vi "test Endpoint Configurations.vi"(8 "error in (no error)":errorcluster, 11 "TestCase in":refnum<class "SLSC Switch Scripting Unit Tests.lvclass">) -> (0 "error out":errorcluster, 3 "TestCase out":refnum<class "SLSC Switch Scripting Unit Tests.lvclass">)   [LabVIEW 2017, in "SLSC Switch Scripting Unit Tests.lvclass"]
uses:
  SLSC Switch Scripting Unit Tests.lvclass
  Endpoint Configuration/Endpoint Configuration Enum.ctl
  SLSC Switch Scripting Unit Tests.lvclass/SLSC Switch Scripting Unit Tests.ctl
  <vilib>/addons/_JKI Toolkits/VI Tester/TestCase.llb/TestCase.lvclass
  SLSC Switch Scripting.lvlib
  C:/Program Files (x86)/National Instruments/LabVIEW 2017/vi.lib/addons/_JKI Toolkits/VI Tester/TestCase.llb/TestCase.lvclass
panel:
  in  "Save?":bool
  out "Output Filename":string
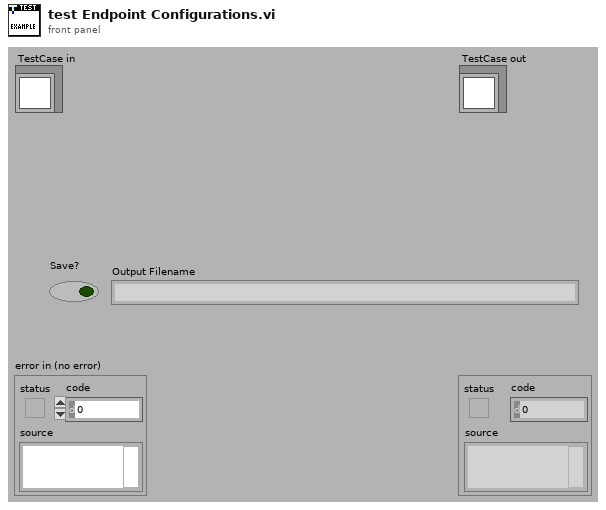
[diagram p1: front panel]
types:
  T1 = typedef "SLSC Switch Scripting.lvlib/Endpoint Configuration Enum.ctl" = enum16{"Load", "Source", "Configuration"}
  T2 = typedef "Custom Device API.lvlib/Custom Device Item Ref.ctl" = u64
  T3 = typedef "SLSC Switch Scripting.lvlib/Endpoint Configuration Cluster.ctl" = cluster{"endpoint":string, "configuration":T1}
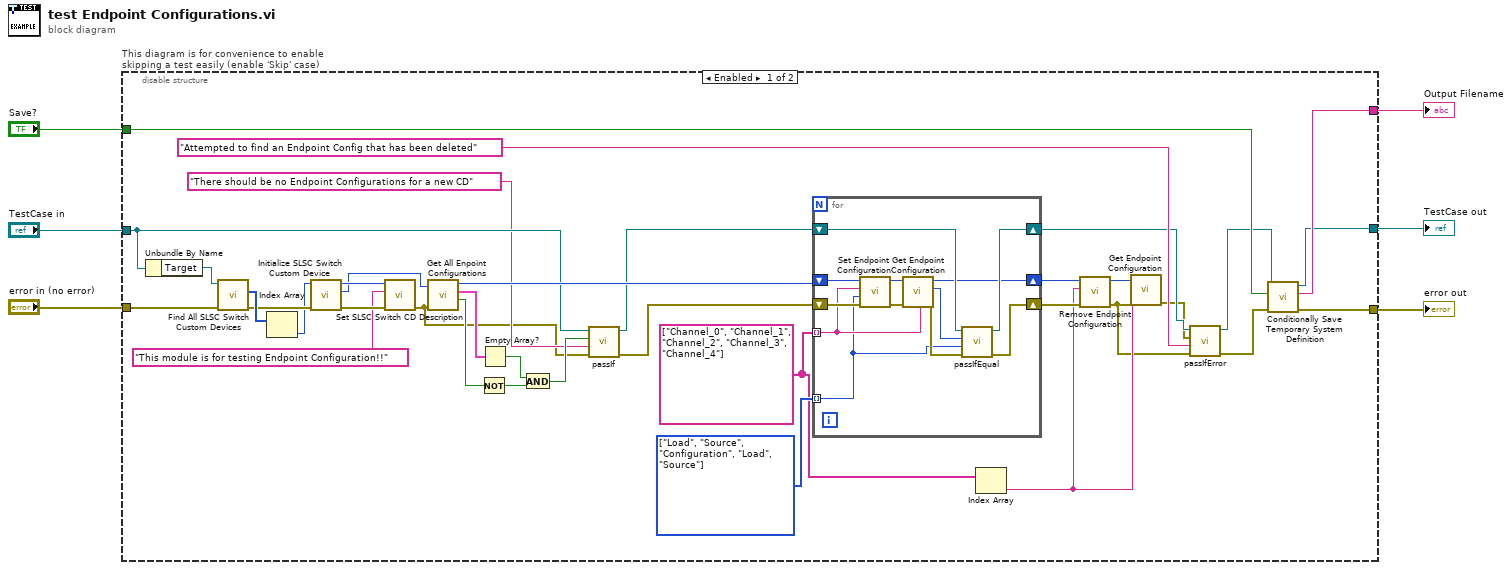
[diagram p0: block diagram]
diagram:
  n1 = disable-structure "This diagram is for convenience to enable skipping a test easily (enable 'Skip' case)" shown="Enabled" {
    disable-tunnel: "TestCase in" -> [w22 w58]
    disable-tunnel: [w40 w56] -> w3
    disable-tunnel: [w41 w57] -> w5
    disable-tunnel: "error in (no error)" -> [w34 w55]
    disable-tunnel: [w42 _] -> w2
    disable-tunnel: "Save?" -> [w39 _]
    frame Enabled {
      w16 = string[] ["Channel_0", "Channel_1", "Channel_2", "Channel_3", "Channel_4"]
      w30 = T1[] [enum."Load", enum."Source", enum."Configuration", enum."Load", enum."Source"] items=["Load", "Source", "Configuration"]
      n2 = Unbundle By Name(w22) -> ("Target"=w35:refnum<k24>)
      n3 = call "Find All SLSC Switch Custom Devices.vi"("error in (no error)"=w34, "Target in"=w35) -> ("error out"=w37:errorcluster, "SLSC Switch Custom Device Ref IDs"=w38:T2[])  [unwired: 7 in, 1 out]
      n4 = Index Array(array=w38) -> (element=w36:T2)  [unwired: 1 in]
      n5 = call "Initialize SLSC Switch Custom Device.vi"("error in (no error)"=w37, "SLSC Sw Custom Device Ref in"=w36) -> ("error out"=w32:errorcluster, "Endpoint Configuration Section Ref"=w29:T2, "SLSC Sw Custom Device Ref out"=w33:T2)  [unwired: 7 in]
      n6 = call "Set SLSC Switch CD Description.vi"("error in (no error)"=w32, "Description"="This module is for testing Endpoint Configuration!!", "SLSC Sw Custom Device Ref in"=w33) -> ("error out"=w18:errorcluster)  [unwired: 7 in, 1 out]
      n7 = call "Get All Enpoint Configurations.vi"("error in (no error)"=w18, "Endpoint Config Section Ref in"=w29) -> ("Endpoints found"=w24:bool, "All Endpoint Configurations"=w27:T3[], "Endpoint Config Section Ref out"=w28:T2)  [unwired: 6 in, 1 out]
      n8 = Not(x=w24) -> (.not. x?=w25:bool)
      n9 = Empty Array?(array=w27) -> (empty?=w26:bool)
      n10 = And(x=w26, y=w25) -> (x .and. y?=w23:bool)
      n11 = call-dynamic "passIf.vi"("error in (no error)"=w18, "message (\"\")"="There should be no Endpoint Configurations for a new CD" ("message (\"\")"), "pass"=w23, "TestCase in"=w22) -> ("error out"=w19:errorcluster, "TestCase out"=w21:refnum<class "SLSC Switch Scripting Unit Tests.lvclass">)  [unwired: 6 in]
      n12 = for {
        shift-right: [w47] -> w15
        shift-left: w19 -> [w53]
        shift-right: [w49] -> w11
        shift-left: w21 -> [w50]
        tunnel: w16 -> [w46] mode=indexing
        tunnel: w30 -> [w43] mode=indexing
        shift-right: [w45] -> w17
        shift-left: w28 -> [w54]
        n13 = call "Set Endpoint Configuration.vi"("error in (no error)"=w53, "Configuration Type"=w43, "Endpoint"=w46, "Endpoint Config Section Ref in"=w54) -> ("error out"=w51:errorcluster, "Endpoint Config Section Ref in"=w52:T2)  [unwired: 6 in]
        n14 = call "Get Endpoint Configuration.vi"("error in (no error)"=w51, "Endpoint"=w46, "Endpoint Config Section Ref in"=w52) -> ("error out"=w48:errorcluster, "Configuration Type"=w44:T1, "Endpoint Config Section Ref out"=w45:T2)  [unwired: 5 in, 1 out]
        n15 = call-dynamic "passIfEqual.vi"("error in (no error)"=w48, "y"=w43, "x"=w44, "TestCase in"=w50) -> ("error out"=w47:errorcluster, "TestCase out"=w49:refnum<class "SLSC Switch Scripting Unit Tests.lvclass">)  [unwired: 6 in]
      }
      n16 = Index Array(array=w16) -> (element=w13:string)  [unwired: 1 in]
      n17 = call "Remove Endpoint Configuration.vi"("error in (no error)"=w15, "Endpoint"=w13, "Endpoint Config Section Ref in"=w17) -> ("error out"=w8:errorcluster, "Endpoint Config Section Ref out"=w14:T2)  [unwired: 6 in, 1 out]
      n18 = call "Get Endpoint Configuration.vi"("error in (no error)"=w8, "Endpoint"=w13, "Endpoint Config Section Ref in"=w14) -> ("error out"=w9:errorcluster)  [unwired: 5 in, 3 out]
      n19 = call-dynamic "passIfError.vi"("error in (no error)"=w8, "task (\"\")"="Attempted to find an Endpoint Config that has been deleted" ("message (\"\")"), "error"=w9, "TestCase in"=w11) -> ("error out"=w7:errorcluster, "TestCase out"=w10:refnum<class "SLSC Switch Scripting Unit Tests.lvclass">)  [unwired: 6 in]
      n20 = call "Conditionally Save Temporary System Definition.vi"("error in (no error)"=w7, "Save?"=w39, "Test Case"=w10) -> ("error out"=w41:errorcluster, "filename"=w42:string, "Test Case"=w40:refnum<class "SLSC Switch Scripting Unit Tests.lvclass">)  [unwired: 6 in]
    }
    frame Disabled {
      # "skip test result while test is under development"
      n21 = call <vilib>:"skip.vi"("error in (no error)"=w55, "TestCase in"=w58) -> ("error out"=w57:errorcluster, "TestCase out"=w56:refnum<class "SLSC Switch Scripting Unit Tests.lvclass">)  [unwired: 8 in]
    }
  }
  "error out" <- w5
  "TestCase out" <- w3
  "Output Filename" <- w2
